vi "IMAGENES_SUB1.vi"(7 "Enum":T2(ring), 9 "Error in":errorcluster, 10 "OPERADORES":T1={"Desplazamiento X"=0.0, "Desplazamiento Y"=500.0, "Giro"=0.0, "ZOOM"=0.0} {"ZOOM" min=0.1 max=10.0 step=0.01 scale=0.1..3.7; "Giro" scale=-360.0..360.0; "Desplazamiento Y" min=-500.0 max=500.0 step=1.0 scale=-200.0..200.0; "Desplazamiento X" min=-500.0 max=500.0 step=1.0 scale=-200.0..200.0}, 11 "IMAGEN 1":path) -> (0 "Error Out":errorcluster, 1 "HISTOGRAMA":dbl[][](graph), 2 "IMAGEN MODIFICADA":picture, 3 "IMAGEN ORIGINAL":picture)   [LabVIEW 2016]
panel:
  in  "Stop Button":bool
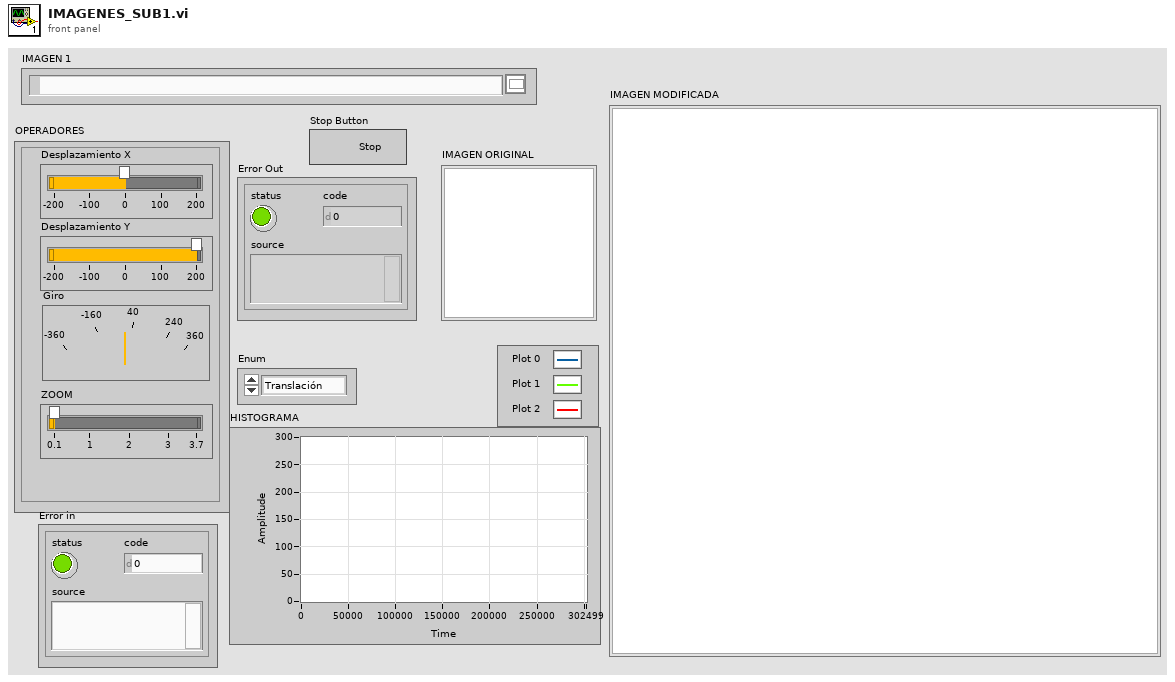
[diagram p1: front panel]
types:
  T1 = cluster{"Desplazamiento X":dbl, "Desplazamiento Y":dbl, "Giro":dbl, "ZOOM":dbl}
  T2 = enum16{"Translación", "Rotación", "Zoom", "GIROH", "GIROV", "Extracción", "Sustitución", "UNION"}
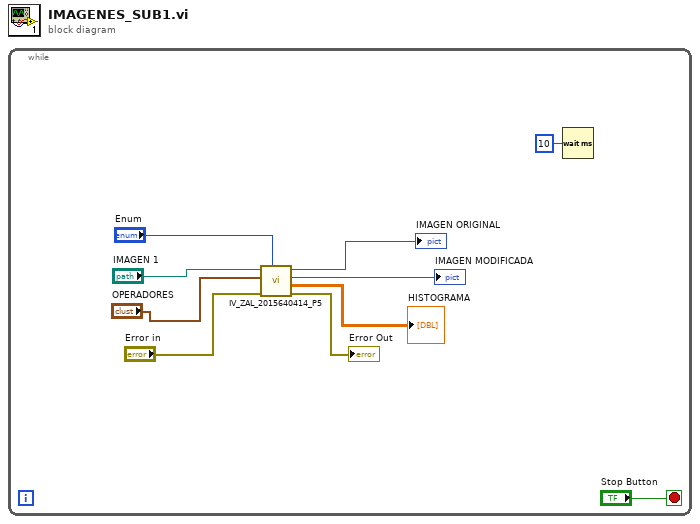
[diagram p0: block diagram]
diagram:
  n1 = while {
    stop <- "Stop Button" stop-if-true
    n2 = call "IV_ZAL_2015640414_P5.vi"("Enum"="Enum", "error in"="Error in", "OPERADORES"="OPERADORES", "IMAGEN 1"="IMAGEN 1") -> ("error out"=→"Error Out":errorcluster, "HISTOGRAMA"=→"HISTOGRAMA":dbl[][], "IMAGEN MODIFICADA"=→"IMAGEN MODIFICADA":picture, "IMAGEN ORIGINAL"=→"IMAGEN ORIGINAL":picture)  [unwired: 4 in]
    n3 = Wait (ms)(milliseconds to wait=u32 10) -> ()  [unwired: 1 out]
  }
